vi "Test Parallell Runner Return one Test Run Result.vi"(8 "error in (no error)":errorcluster, 11 "Test Runner Test in":refnum<class "Test Runner Test.lvclass">) -> (0 "error out":errorcluster, 3 "Test Runner Test out":refnum<class "Test Runner Test.lvclass">)   [LabVIEW 2020, in "Test Runner Test.lvclass"]
uses:
  Test Runner Test.lvclass
  C:/git/astemes-lunit/source/Framework/Result Observer/Result Observer.lvclass
  source/Framework/Parallell Test Runner/Parallell Test Runner.lvclass
  source/API/LUnit Test Suite/LUnit Test Suite.lvclass
  C:/git/astemes-lunit/source/Core/Runnable/Runnable.lvclass
  Test Runner Test.lvclass/Test Runner Test.ctl
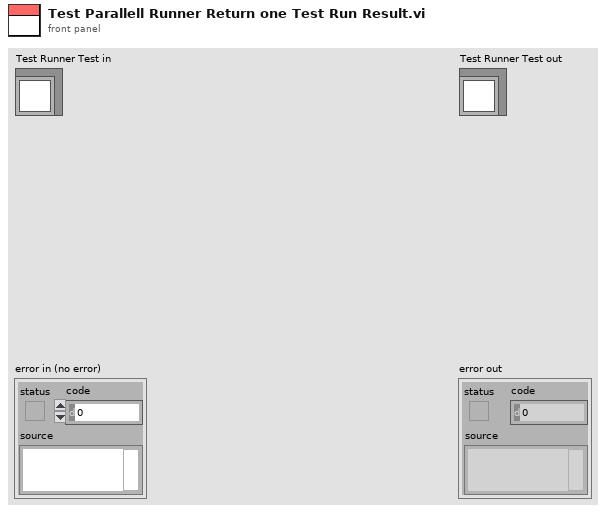
[diagram p1: front panel]
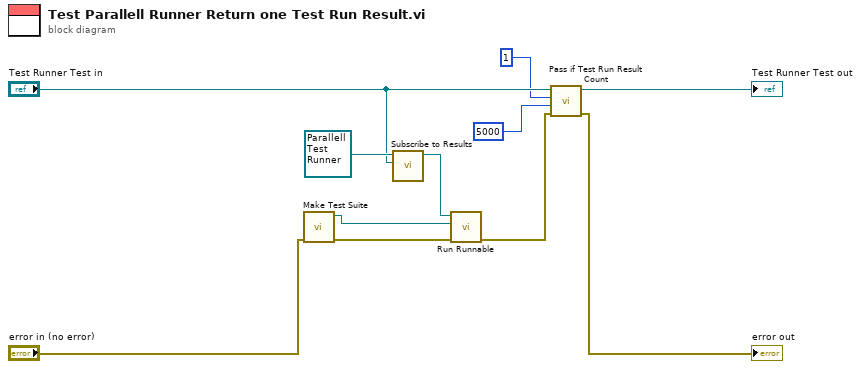
[diagram p0: block diagram]
diagram:
  n1 = call "Make Test Suite.vi"("error in (no error)"="error in (no error)") -> ("error out"=w10:errorcluster, "LUnit Test Suite V2 out"=w11:refnum<class "LUnit Test Suite.lvclass">)  [unwired: 9 in]
  n2 = call-dynamic "Subscribe to Results.vi"("Result Observer"="Test Runner Test in", "Parallell Test Runner In"=refnum<class "Parallell Test Runner.lvclass"> refnum ("Test Runner")) -> ("Parallell Test Runner Out"=w3:refnum<class "Parallell Test Runner.lvclass">)  [unwired: 8 in, 1 out]
  n3 = call-dynamic "Run Runnable.vi"("error in (no error)"=w10, "Runnable"=w11, "Parallell Test Runner In"=w3) -> ("error out"=w8:errorcluster)  [unwired: 7 in, 1 out]
  n4 = call "Pass if Test Run Result Count.vi"("error in (no error)"=w8, "timeout in ms (0)"=5000, "Required Number of Suite Results"=1, "Test Runner Test in"="Test Runner Test in") -> ("error out"=→"error out":errorcluster, "Test Runner Test out"=→"Test Runner Test out":refnum<class "Test Runner Test.lvclass">)  [unwired: 6 in]
